vi "test.ini_to_object.vi"() -> ()   [LabVIEW 2020]
uses:
  configuration-data/configuration-data.lvclass/configuration-data.ctl
  500ea461-7ed1-4b27-9855-0b724d609ef0.vi
  configuration-data/configuration.get.vi
  configuration-data/configuration.set.vi
  <vilib>/addons/_JKI.lib/_jki_lib_configuration_file.llb/Open Config String__jki_lib_configuration_file.vi
  <vilib>/Utility/config.llb/Get Section Names.vi
  <vilib>/Utility/config.llb/Get Key Names.vi
  <vilib>/Utility/config.llb/Read Key.vi
  <vilib>/Utility/config.llb/Read Key (String).vi
  configuration-data/datatype_conversion.vi
  <vilib>/Utility/config.llb/Close Config Data.vi
  <vilib>/addons/_JKI Toolkits/Caraya/classes/Assert/Assert Not Error.vi
  <vilib>/addons/_JKI Toolkits/Caraya/classes/Assert/Assert Equal Value_Variant.vi
  configuration-data/configuration-data.lvclass
  <vilib>/regexp/Match Regular Expression.xnode
  toml/toml.lvclass
  <vilib>/addons/_JKI Toolkits/Caraya/classes/Test/Test.lvclass
  <vilib>/addons/_JKI Toolkits/Caraya/classes/Assert/Assert.lvclass
  69a6e8de-393c-4c9f-9cb0-378016c2121b.vi
  3b4e3ec6-e3cf-40c1-b630-d128edea10dd.vi
panel:
  out "Map":map{string, map{string, string}}(c390)
  out "toml":string
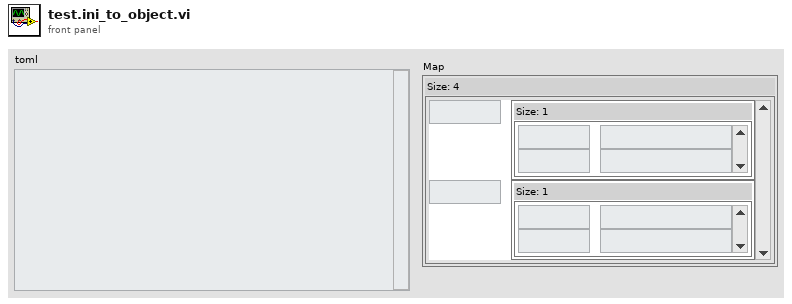
[diagram p1: front panel]
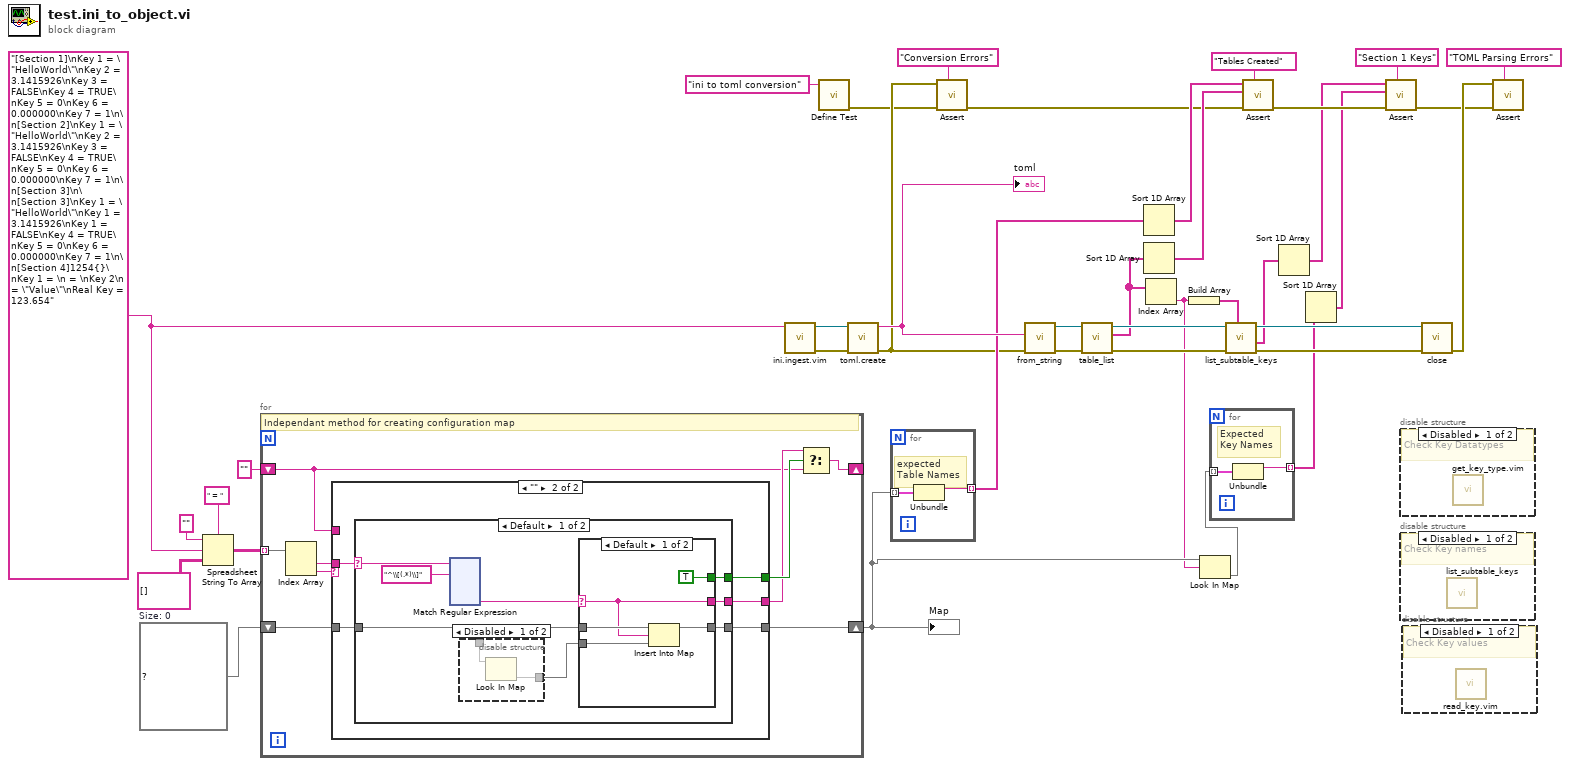
[diagram p0: block diagram]
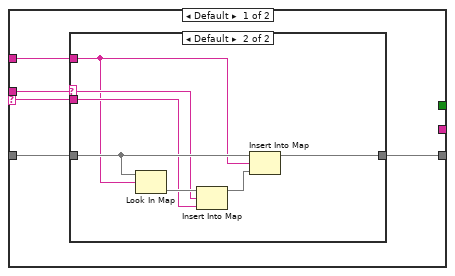
[diagram p5: hidden frame]
diagram:
  w26 = map{string, map{string, string}} {}  # Size: 0
  w1 = "[Section 1]\nKey 1 = \"HelloWorld\"\nKey 2 = 3.1415926\nKey 3 = FALSE\nKey 4 = TRUE\nKey 5 = 0\nKey 6 = 0.000000\nKey 7 = 1\n\n[Section 2]\nKey 1 = \"HelloWorld\"\nKey 2 = 3.1415926\nKey 3 = FALSE\nKey 4 = TRUE\nKey 5 = 0\nKey 6 = 0.000000\nKey 7 = 1\n\n[Section 3]\n\n[Section 3]\nKey 1 = \"HelloWorld\"\nKey 1 = 3.1415926\nKey 1 = FALSE\nKey 4 = TRUE\nKey 5 = 0\nKey 6 = 0.000000\nKey 7 = 1\n\n[Section 4]1254{}\nKey 1 = \n = \nKey 2\n = \"Value\"\nReal Key = 123.654" ("config string or path")
  n1 = Spreadsheet String To Array(delimiter (Tab)=" = ", format string="", spreadsheet string=w1, array type (2D Dbl)=string[][] []) -> (array=w28:string[][])
  n2 = for {
    tunnel: w28 -> [w48] mode=indexing
    shift-right: [w44] -> w11
    shift-left: w26 -> [w45]
    shift-right: [w41] -> _
    shift-left: "" -> [w40]
    # "Independant method for creating configuration map"
    n3 = Index Array(array=w48) -> (element #1=w46:string, element #2=w47:string)  [unwired: 2 in]
    n4 = case shown="\"\"" w47 {
      selector: w47 -> [w49 _]
      tunnel: w46 -> [w53 w66]
      tunnel: w45 -> [w50 w65]
      tunnel: [w51 w64] -> w44
      tunnel: [_ w63] -> w42
      tunnel: [_ w62] -> w43
      tunnel: w40 -> [w52 _]
      frame Default {
        n5 = case shown="Default" w53 {
          selector: w53 -> [_ w57]
          tunnel: w52 -> [_ w56]
          tunnel: [w54 w60] -> w51
          tunnel: w50 -> [w54 w61]
          tunnel: w49 -> [_ w58]
          frame "" {
          }
          frame Default {
            n6 = Look In Map(map=w61, key=w56) -> (value=w59:map{string, string})  [unwired: 1 in, 1 out]
            n7 = Insert Into Map(map in=w59, key=w57, value=w58) -> (map out=w55:map{string, string})  [unwired: 2 out]
            n8 = Insert Into Map(map in=w61, key=w56, value=w55) -> (map out=w60:map{string, map{string, string}})  [unwired: 2 out]
          }
        }
      }
      frame "" {
        n9 = case shown="Default" w66 {
          selector: w66 -> [w73 _]
          tunnel: w65 -> [w68 w199]
          tunnel: [w71 w199] -> w64
          tunnel: [w70 _] -> w63
          tunnel: [w69 _] -> w62
          frame Default {
            n10 = xnode "Match Regular Expression"("input string"=w73, "regular expression"="^\\[(.*)\\]") -> ("submatch 1"=w72:string)  [unwired: 4 in, 5 out]
            n11 = disable-structure shown="Disabled" {
              disable-tunnel: w68 -> [w76 _]
              disable-tunnel: [w75 _] -> w67
              frame Disabled {
                n12 = Look In Map(map=w76) -> (value=w75:map{string, string})  [unwired: 2 in, 1 out]
              }
              frame Enabled {
              }
            }
            n13 = case shown="Default" w72 {
              selector: w72 -> [w78 _]
              tunnel: w68 -> [w81 w82]
              tunnel: [w80 w82] -> w71
              tunnel: [w78 _] -> w70
              tunnel: [TRUE _] -> w69
              tunnel: w67 -> [w77 _]
              frame Default {
                n14 = Insert Into Map(map in=w81, key=w78, value=w77) -> (map out=w80:map{string, map{string, string}})  [unwired: 2 out]
              }
              frame "" {
              }
            }
          }
          frame "" {
          }
        }
      }
    }
    n15 = Select(t=w42, s=w43, f=w40) -> (s? t:f=w41:string)
  }
  "Map" <- w11
  n16 = call "ini.ingest.vim"("config string or path"=w1) -> ("error out"=w38:errorcluster, "configuration-data"=w39:refnum<class "configuration-data.lvclass">)  [unwired: 9 in]
  n17 = call <vilib>:"Define Test.vi"("Label (VI Title)"="ini to toml conversion") -> ("error out"=w22:errorcluster)  [unwired: 10 in]
  n18 = call "toml.create.vi"("error in"=w38, "configuration-data"=w39) -> ("error out"=w23:errorcluster, "toml"=w37:string)  [unwired: 8 in]
  "toml" <- w37
  n19 = for {
    tunnel: w11 -> [w201] mode=indexing
    tunnel: [w200] -> w24 mode=indexing
    # "expected\nTable Names"
    n20 = Unbundle(w201) -> (w200:string)  [unwired: 1 out]
  }
  n21 = call-poly <vilib>:"Assert.vi"("Label"="Conversion Errors", "error in (no error)"=w22, "Not Error?"=w23) -> ("error out"=w21:errorcluster)  [unwired: 8 in]
  n22 = call "from_string.vi"("error in (no error)"=w23, "toml"=w37) -> ("error out"=w35:errorcluster, "toml out"=w36:refnum<class "toml.lvclass">)  [unwired: 8 in]
  n23 = call "table_list.vi"("error in (no error)"=w35, "toml in"=w36) -> ("error out"=w15:errorcluster, "tables"=w13:string[], "toml out"=w17:refnum<class "toml.lvclass">)  [unwired: 7 in]
  n24 = Sort 1D Array(array=w24) -> (sorted array=w33:string[])
  n25 = Sort 1D Array(array=w13) -> (sorted array=w32:string[])
  n26 = Index Array(array=w13) -> (element=w10:string)  [unwired: 1 in]
  n27 = Build Array(w10) -> (w12:string[])
  n28 = Look In Map(map=w11, key=w10) -> (value=w9:map{string, string})  [unwired: 1 in, 1 out]
  n29 = for {
    tunnel: w9 -> [w203] mode=indexing
    tunnel: [w202] -> w4 mode=indexing
    # "Expected\nKey Names"
    n30 = Unbundle(w203) -> (w202:string)  [unwired: 1 out]
  }
  n31 = call "list_subtable_keys.vi"("subtables"=w12, "error in (no error)"=w15, "toml in"=w17) -> ("error out"=w14:errorcluster, "keys"=w5:string[], "toml out"=w16:refnum<class "toml.lvclass">)  [unwired: 5 in, 1 out]
  n32 = call-poly <vilib>:"Assert.vi"("Label"="Tables Created", "error in (no error)"=w21, "Y"=w32, "X"=w33) -> ("error out"=w7:errorcluster)  [unwired: 7 in]
  n33 = Sort 1D Array(array=w5) -> (sorted array=w3:string[])
  n34 = Sort 1D Array(array=w4) -> (sorted array=w2:string[])
  n35 = call-poly <vilib>:"Assert.vi"("Label"="Section 1 Keys", "error in (no error)"=w7, "Y"=w2, "X"=w3) -> ("error out"=w6:errorcluster)  [unwired: 7 in]
  n36 = disable-structure shown="Disabled" {
    frame Disabled {
      # "Check Key Datatypes"
      n37 = call "get_key_type.vim"() -> ()  [unwired: 7 in, 5 out]
    }
    frame Enabled {
    }
  }
  n38 = disable-structure shown="Disabled" {
    frame Disabled {
      # "Check Key names"
      n39 = call "list_subtable_keys.vi"() -> ()  [unwired: 8 in, 4 out]
    }
    frame Enabled {
    }
  }
  n40 = disable-structure shown="Disabled" {
    frame Disabled {
      # "Check Key values"
      n41 = call "read_key.vim"() -> ()  [unwired: 8 in, 4 out]
    }
    frame Enabled {
    }
  }
  n42 = call "close.vi"("error in (no error)"=w14, "toml in"=w16) -> ("error out"=w18:errorcluster)  [unwired: 9 in]
  n43 = call-poly <vilib>:"Assert.vi"("Label"="TOML Parsing Errors", "error in (no error)"=w6, "Not Error?"=w18) -> ()  [unwired: 8 in, 1 out]
